vi "Start HTTP.vi"(8 "error in (no error)":errorcluster, 11 "Vecto in":refnum<class "Vecto.lvclass">) -> (0 "error out":errorcluster, 3 "Vecto out":refnum<class "Vecto.lvclass">)   [LabVIEW 2020, in "Vecto.lvlib" / "Vecto.lvclass"]
uses:
  Vecto.lvclass
  Vecto.lvclass/Vecto.ctl
  Connection Info.ctl
  Connection Type.ctl
  proto/ServiceType/Enumeration.ctl
  <vilib>/IlluminatedG/IG HTTP Server/HTTP Server/Server/Server.lvclass
  Node Config/Node Config.lvclass
  Vecto.lvlib
  VectoService/VectoInfo.lvclass
  NodeDiscovery/NodeDiscovery.lvclass
  proto/ServiceType/ServiceType.lvlib
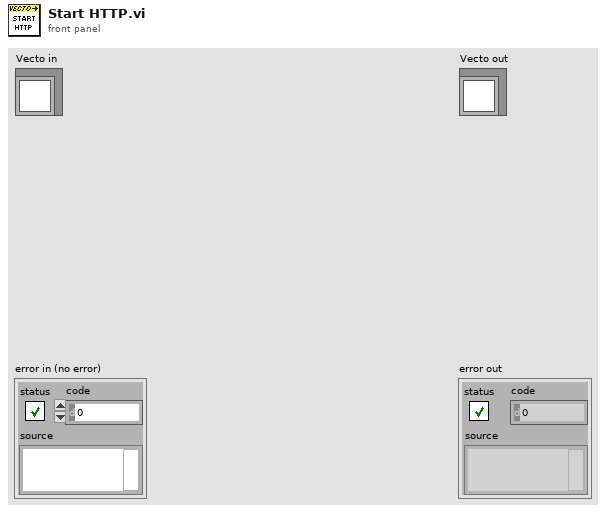
[diagram p1: front panel]
types:
  T1 = typedef "ServiceType.lvlib/Enumeration.ctl" = enum16{"SERVICETYPE_UNKNOWN", "SERVICETYPE_TCPSERVER", "SERVICETYPE_HTTPSERVER"}
  T2 = typedef "Vecto.lvlib/Connection Type.ctl" = enum16{"TCP", "Telemetry", "Discovery", "HTTP"}
  T3 = typedef "Vecto.lvlib/Connection Info.ctl" = cluster{"Name":string, "Type":T2, "RXCount":i32, "TXCount":i32, "Connected":bool, "RemoteIP":u32, "RemotePort":u16, "LocalPort":u16}
  T4 = typedef "Vecto.lvlib/Node Config.lvclass/HTTP Server Info.ctl" = cluster{"HTTP Port":u16, "Debug":bool}
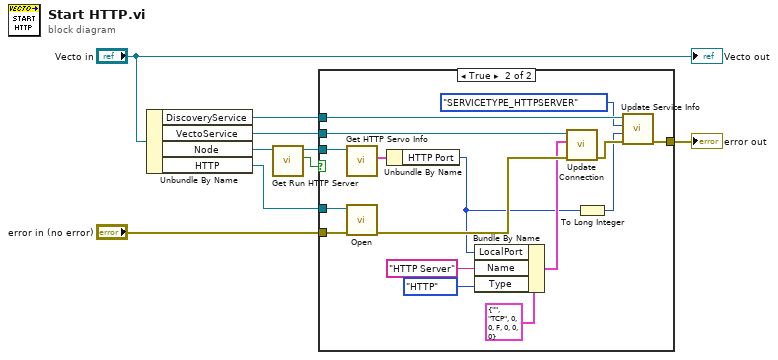
[diagram p0: block diagram]
diagram:
  n1 = Unbundle By Name("Vecto in") -> ("DiscoveryService"=w7:refnum<class "NodeDiscovery.lvclass">, "VectoService"=w8:refnum<class "VectoInfo.lvclass">, "Node"=w4:refnum<class "Node Config.lvclass">, "HTTP"=w1:refnum<class "Server.lvclass">)
  n2 = call "Get Run HTTP Server.vi"("Node Config in"=w4) -> ("Run HTTP Server"=w2:bool, "Node Config out"=w3:refnum<class "Node Config.lvclass">)  [unwired: 8 in, 1 out]
  n3 = case shown="True" w2 {
    tunnel: "error in (no error)" -> [w10 w24]
    tunnel: w8 -> [_ w19]
    tunnel: w7 -> [_ w18]
    tunnel: [w10 w17] -> w6
    tunnel: w3 -> [_ w14]
    tunnel: w1 -> [_ w13]
    frame False {
    }
    frame True {
      n4 = call "Get HTTP Servo Info.vi"("Node in"=w14) -> ("HTTP Server Info"=w16:T4)  [unwired: 8 in, 2 out]
      n5 = call <vilib>:"Open.vi"("error in (no error)"=w24, "Server in"=w13) -> ("error out"=w25:errorcluster)  [unwired: 8 in, 1 out]
      n6 = Unbundle By Name(w16) -> ("HTTP Port"=w15:u16)
      n7 = Bundle By Name(cluster=T3 {"Name"="", "Type"=enum."TCP", "RXCount"=0, "TXCount"=0, "Connected"=FALSE, "RemoteIP"=0, "RemotePort"=0, "LocalPort"=0} ("Connection Info"), "LocalPort"=w15, "Name"="HTTP Server", "Type"=Connection_Type."HTTP") -> (w20:T3)
      n8 = call "Update Connection.vi"("error in (no error)"=w25, "Connection Info"=w20, "VectoService in"=w19) -> ("error out"=w26:errorcluster)  [unwired: 7 in, 1 out]
      n9 = To Long Integer(number=w15) -> (32bit integer=w11:i32)
      n10 = call "Update Service Info.vi"("error in (no error)"=w26, "Port"=w11, "Type"=Enumeration."SERVICETYPE_HTTPSERVER" ("type"), "DiscoveryService in"=w18) -> ("error out"=w17:errorcluster)  [unwired: 6 in, 1 out]
    }
  }
  "error out" <- w6
  "Vecto out" <- "Vecto in"
